vi "GetPhasorByChannelName.vi"(8 "error in (no error)":errorcluster, 10 "Channel Name":string, 11 "Channels Phasor":T1[](array[typedef])) -> (0 "error out":errorcluster, 1 "Channel Phasor":T1, 2 "Found?":bool)   [LabVIEW 2017, in "McsaUtilities.lvlib"]
uses:
  <vilib>/addons/InsightCM/Utilities/Analysis/MCSA/controls/McsaChannelPhasor.ctl
  <vilib>/addons/InsightCM/Utilities/MCSA/McsaUtilities.lvlib
  <vilib>/addons/InsightCM/Utilities/Analysis/MCSA/McsaAnalysisFunctions.lvlib
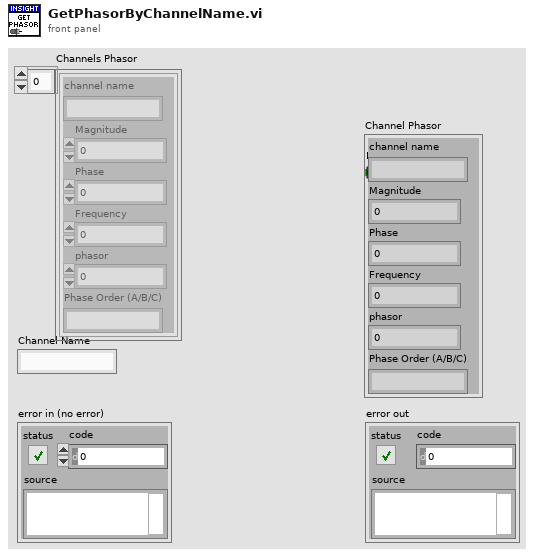
[diagram p1: front panel]
types:
  T1 = typedef "McsaAnalysisFunctions.lvlib/McsaChannelPhasor.ctl" = cluster{"channel name":string, "Magnitude":dbl, "Phase":dbl, "Frequency":dbl, "phasor":cdb, "Phase Order (A/B/C)":string}
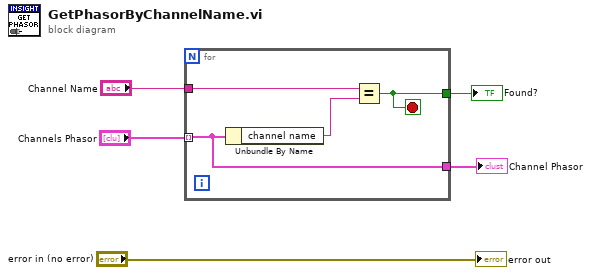
[diagram p0: block diagram]
diagram:
  n1 = for {
    tunnel: "Channels Phasor" -> [w6] mode=indexing
    tunnel: "Channel Name" -> [w9]
    tunnel: [w8] -> w4
    tunnel: [w6] -> w1
    stop <- w8 stop-if-true
    n2 = Unbundle By Name(w6) -> ("channel name"=w7:string)
    n3 = Equal?(x=w9, y=w7) -> (x = y?=w8:bool)
  }
  "Found?" <- w4
  "Channel Phasor" <- w1
  "error out" <- "error in (no error)"
